vi "thermo_check_valid_units_all.vi"() -> (0 "valids count":i16, 1 "valids 2D":bool[][](array[boolean]), 2 "valids":bool[](array[boolean]))   [LabVIEW 2020]
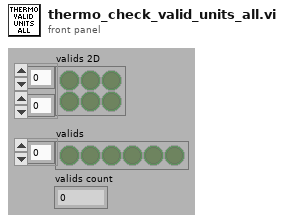
[diagram p1: front panel]
types:
  T1 = typedef "thermo.ctl" = cluster{"stat":enum16{"Disabled", "Enabled"}, "type":T2, "comment":string, "tag":string, "refresh":dbl, "IP":string, "port":u16, "VISA":refnum<visa-resource-name>, "last readout":timestamp, "TCP ref":refnum<k5>, "VISA sess":refnum<visa-resource-name>, "idn":string, "press":dbl, "RH":dbl, "temp":dbl, "pres cor":dbl[][], "RH cor":dbl[][], "temp cor":dbl[][], "try left":i32, "failed":bool, "RTD set":dbl[], "RTD inv":dbl[], "range":dbl, "net mode":enum16{"MODBUS", "HTTP"}, "try fail":T3, "timeout [s]":dbl, "max retries":i32}
  T2 = typedef "thermo_types.ctl" = enum16{"Disabled", "Simulated", "COMET Tx5xx (ethernet)", "Keithley 2002 (GPIB) + RTD", "Agilent 344xx (GPIB) + RTD"}
  T3 = typedef "Thermometer Fail Action.ctl" = enum16{"Stop trying - keep last value", "Stop trying - return NaN", "Generate error - stop sweep"}
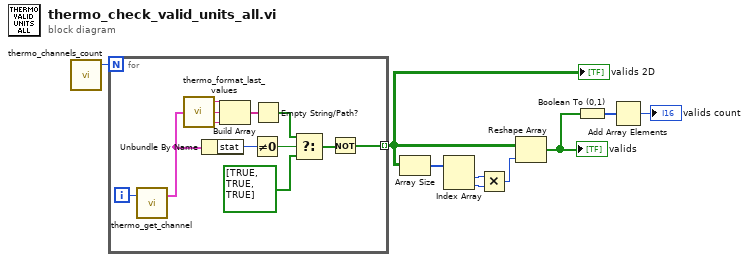
[diagram p0: block diagram]
diagram:
  n1 = call "thermo_channels_count.vi"() -> ("channels"=w9:i32)  [unwired: 2 in]
  n2 = for {
    N: w9 -> [_]
    tunnel: [w11] -> w4 mode=indexing
    i -> [w21]
    n3 = call "thermo_get_channel.vi"("index"=w21) -> ("channel"=w10:T1)  [unwired: 1 in, 1 out]
    n4 = call "thermo_format_last_values.vi"("thermo"=w10) -> ("temperature"=w18:string, "RH"=w20:string, "pressure"=w19:string)  [unwired: 4 in]
    n5 = Unbundle By Name(w10) -> ("stat"=w17:enum16{"Disabled", "Enabled"})
    n6 = Build Array(w18, w20, w19) -> (w15:string[])
    n7 = Not Equal To 0?(x=w17) -> (x != 0?=w16:bool)
    n8 = Empty String/Path?(string/path=w15) -> (empty?=w14:bool[])
    n9 = Select(t=w14, s=w16, f=bool[] [TRUE, TRUE, TRUE]) -> (s? t:f=w13:bool[])
    n10 = Not(x=w13) -> (.not. x?=w11:bool[])
  }
  "valids 2D" <- w4
  n11 = Array Size(array=w4) -> (size(s)=w8:i32[])
  n12 = Index Array(array=w8) -> (element #1=w6:i32, element #2=w7:i32)  [unwired: 2 in]
  n13 = Multiply(x=w6, y=w7) -> (x*y=w5:i32)
  n14 = Reshape Array(w4, w5) -> (w3:bool[])
  "valids" <- w3
  n15 = Boolean To (0,1)(Boolean=w3) -> (0, 1=w2:i16[])
  n16 = Add Array Elements(numeric array=w2) -> (sum=→"valids count":i16)
